vi "One-hot_sub.vi"(1 "Input(Y)":i32) -> (0 "Output(One-hot)":i32[](array[numeric]))   [LabVIEW 2021]
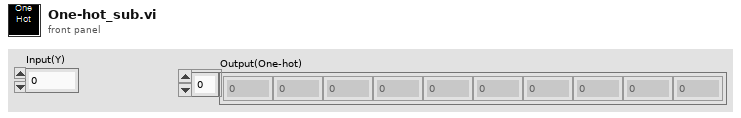
[diagram p1: front panel]
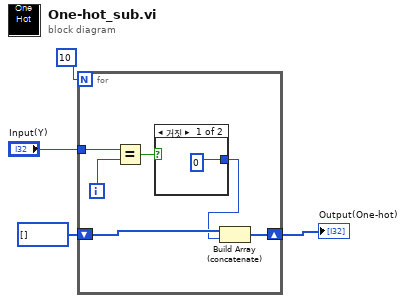
[diagram p0: block diagram]
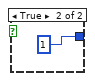
[diagram p2: hidden frame]
diagram:
  n1 = for {
    N: 10 ("No.Class") -> [_]
    shift-right: [w9] -> w2
    shift-left: i32[] [] -> [w10]
    tunnel: "Input(Y)" -> [w7]
    i -> [w6]
    n2 = Equal?(x=w7, y=w6) -> (x = y?=w8:bool)
    n3 = case shown="거짓" w8 {
      tunnel: [0 1] -> w5
      frame False {
      }
      frame True {
      }
    }
    n4 = Build Array (concatenate)(w10, w5) -> (w9:i32[])
  }
  "Output(One-hot)" <- w2
